vi "macro_SlewRateLimter_Execute.vi"   [LabVIEW 2019, in "Trajectory_Library.lvlib"]
uses:
  Trajectory_Library.lvlib
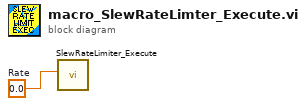
[diagram p0: block diagram]
diagram:
  w1 = 0.0  # Rate
  n1 = call "SlewRateLimiter_Execute.vi"("PositiveRate"=w1) -> ()  [unwired: 9 in, 2 out]
